vi "executeCommand.vi"(8 "error in (no error)":errorcluster, 9 "input":variant, 10 "commands":T2, 11 "AlCS in":refnum<class "AlCS.lvclass">) -> (0 "error out":errorcluster, 1 "value":variant, 2 "data":T1, 3 "AlCS out":refnum<class "AlCS.lvclass">)   [LabVIEW 2016, in "AlCS.lvclass"]
uses:
  AlCS.lvclass
  Typedefs/Commands.ctl
  Typedefs/data.ctl
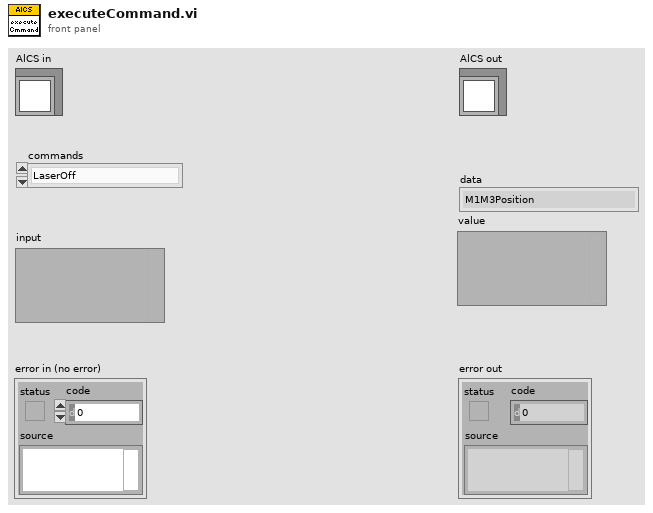
[diagram p1: front panel]
types:
  T1 = typedef "data.ctl" = enum16{"M1M3Position", "M2Position", "CameraPosition", "LaserStatus", "DeviceStatus", "Ack"}
  T2 = typedef "Commands.ctl" = enum16{"LaserOff", "MP", "queryStatus", "queryLaserStatus", "queryPosition", "clearError"}
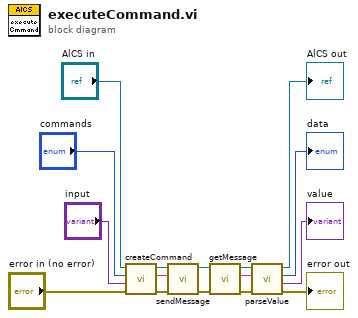
[diagram p0: block diagram]
diagram:
  n1 = call "createCommand.vi"("error in (no error)"="error in (no error)", "Variant"="input", "commands"="commands", "AlCS in"="AlCS in") -> ("error out"=w11:errorcluster, "command"=w4:string, "AlCS out"=w16:refnum<class "AlCS.lvclass">)  [unwired: 5 in]
  n2 = call "sendMessage.vi"("error in (no error)"=w11, "message"=w4, "AlCS in"=w16) -> ("error out"=w10:errorcluster, "AlCS out"=w15:refnum<class "AlCS.lvclass">)  [unwired: 7 in]
  n3 = call "getMessage.vi"("error in (no error)"=w10, "AlCS in"=w15) -> ("error out"=w9:errorcluster, "message"=w3:string, "AlCS out"=w14:refnum<class "AlCS.lvclass">)  [unwired: 7 in]
  n4 = call "parseValue.vi"("error in (no error)"=w9, "message"=w3, "AlCS in"=w14) -> ("error out"=→"error out":errorcluster, "value"=→"value":variant, "data"=→"data":T1, "AlCS out"=→"AlCS out":refnum<class "AlCS.lvclass">)  [unwired: 5 in]
